vi "MagBoard_Processor.vi"() -> ()   [LabVIEW 2018]
uses:
  <vilib>/Math Plots/3D Math Plots/3D Surface/3D Surface XCtrl/3D Surface.xctl
  <vilib>/Math Plots/3D Math Plots/3D Surface/3D Surface Datatype/3D Surface Datatype.lvclass
  subVIs/calibration/FGVs/FGV States.ctl
  <vilib>/Utility/file.llb/Write Delimited Spreadsheet (DBL).vi
  <vilib>/Math Plots/3D Math Plots/3D Surface/3D Surface Datatype/Public/Plot Helper (Matrix).vi
panel:
  out "Node XYZ List":dbl[][](array[numeric])
  out "dT":u32=4294745741
  in  "Calibration File":string="6x0-5mm"
  in  "Save Data":bool=TRUE
  in  "Export File (CSV)":path=path "C:/Users/menprc/Documents/GitHub/MagLib/MagBoard_n64_UI/MagBoard_n64_UI_LabVIEW_Client/example_data/M064_008.csv"
  in  "dT":u32=10
  in  "Tare":bool
  out "Time":u32=4294745741
  in  "stop":bool
  in  "Data File":path=path "C:/Users/menprc/Documents/GitHub/MagLib/MagBoard_n64_UI/MagBoard_n64_UI_LabVIEW_Client/example_data/M064_008_up.dat"
  out "Instantaneous Data":refnum<class "3D Plot Datatype.lvclass">[](xcontrol)
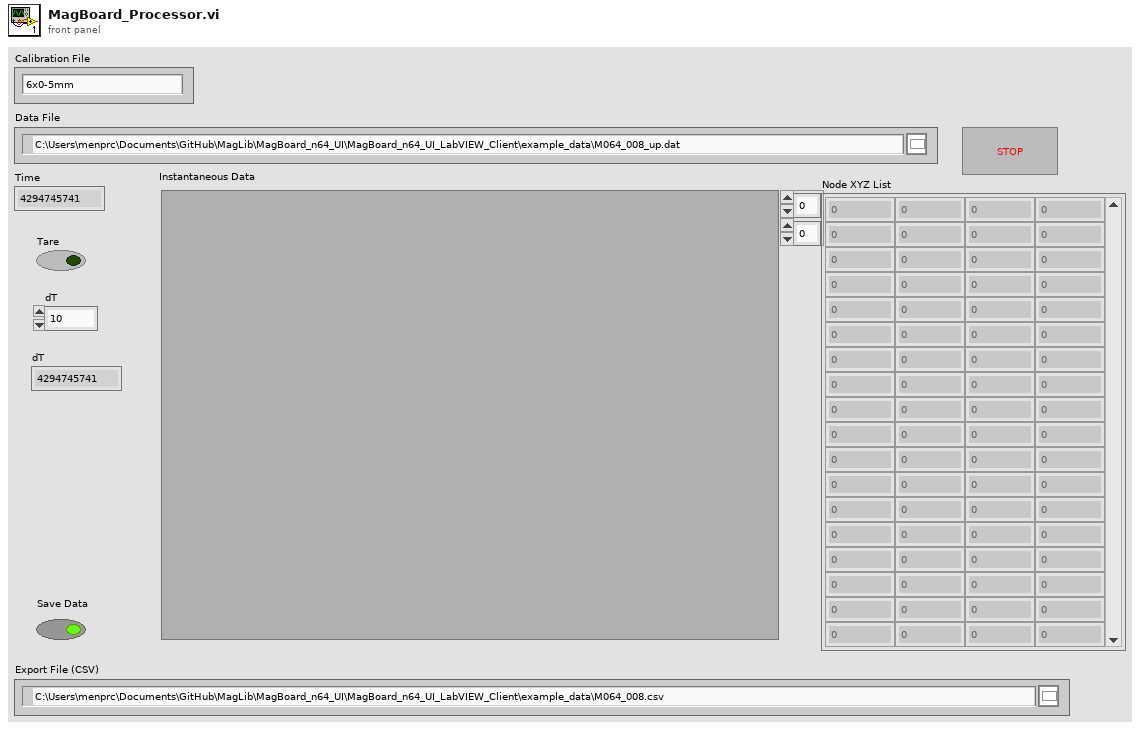
[diagram p1: front panel]
types:
  T1 = typedef "FGV States.ctl" = enum16{"Get", "Set", "Reset"}
  T2 = cluster{cluster{dbl[][], "Array":dbl[][]}, cluster{dbl[][], "Array":dbl[][]}, cluster{dbl[][], "Array":dbl[][]}, cluster{dbl[][], "Array":dbl[][]}}
  T3 = cluster{cluster{dbl[][], "Array":dbl[][]}, cluster{dbl[][], "Array":dbl[][]}, cluster{dbl[][], "Array":dbl[][]}, cluster{dbl[][], "Array":dbl[][]}}[]
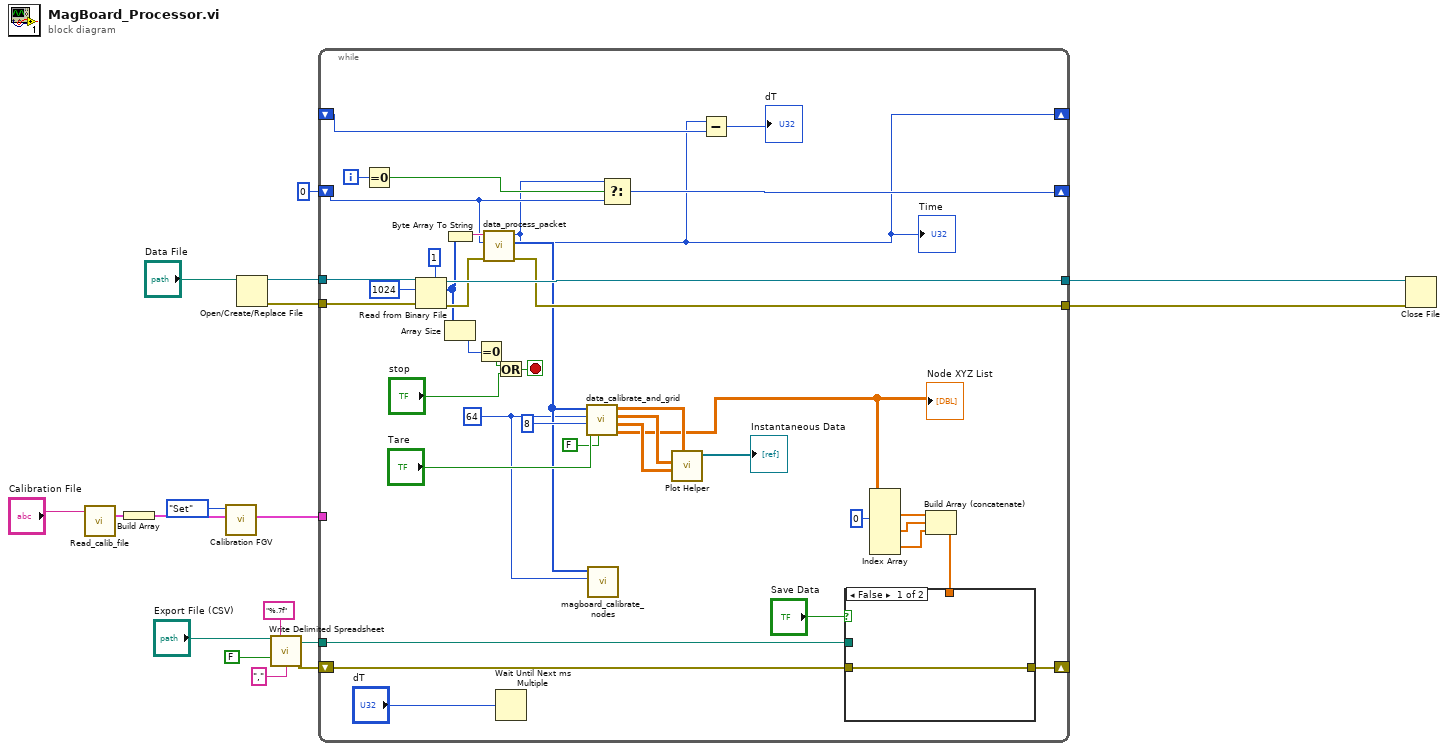
[diagram p0: block diagram]
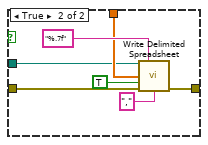
[diagram p2: hidden frame]
diagram:
  n1 = call "Read_calib_file.vi"("string"="Calibration File") -> ("output cluster"=w4:T2)  [unwired: 6 in, 4 out]
  n2 = Build Array(w4) -> (w3:T3)
  n3 = call "Calibration FGV.vi"("Calib in"=w3, "FGV States"=FGV_States."Set") -> ("Calib in 2"=w1:T3)  [unwired: 9 in]
  n4 = Open/Create/Replace File(file path (use dialog)="Data File") -> (refnum out=w16:refnum<file>, error out=w15:errorcluster)  [unwired: 5 in, 1 out]
  n5 = call-poly <vilib>:"Write Delimited Spreadsheet.vi"("file path (dialog if empty)"="Export File (CSV)", "format (%.3f)"="%.7f", "append to file? (new file:F)"=FALSE, "delimiter (\\t)"="," ("delimiter (\\t)")) -> ("new file path (Not A Path if cancelled)"=w8:path, "error out"=w6:errorcluster)  [unwired: 10 in]
  n6 = while {
    tunnel: w16 -> [w57]
    tunnel: w15 -> [w56]
    tunnel: [w54] -> w13
    tunnel: [w49] -> w14
    shift-right: [w48] -> _
    shift-left: u32 0 ("Time") -> [w46]
    tunnel: w8 -> [w32]
    shift-right: [w30] -> _
    shift-left: w6 -> [w31]
    tunnel: w1 -> [_]
    shift-right: [w19] -> _
    shift-left: _ -> [w20]
    i -> [w47]
    stop <- w25 stop-if-true
    w21 = 64 ("No. Nodes")
    n7 = Equal To 0?(x=w47) -> (x = 0?=w42:bool)
    n8 = Read from Binary File(5:u8 1 ("count (1)"), 8:w56, 10:1024 ("count (1)"), 11:w57) -> (0:w50:errorcluster, 2:w28:u8[], 3:w54:refnum<file>)  [unwired: 2 in, 1 out]
    n9 = Byte Array To String(unsigned byte array=w28) -> (string=w51:string)
    n10 = Array Size(array=w28) -> (size(s)=w27:i32)
    n11 = Equal To 0?(x=w27) -> (x = 0?=w26:bool)
    n12 = call "data_process_packet.vi"("error in (no error)"=w50, "No. Sensors"=w46, "Binary Input Data"=w51) -> ("error out"=w49:errorcluster, "Raw Sensors (Flattened)"=w22:i16[], "Time"=w19:u32)  [unwired: 4 in, 2 out]
    "Time" <- w19
    n13 = Or(x=w26, y="stop") -> (x .or. y?=w25:bool)
    n14 = Wait Until Next ms Multiple(millisecond multiple="dT") -> ()  [unwired: 1 out]
    n15 = call "data_calibrate_and_grid.vi"("Reset"=FALSE, "Tare"="Tare", "Row Length"=8, "No. Nodes"=w21, "Sensor Readings (PACKET)"=w22) -> ("Node XYZ List"=w23:dbl[][], "Y (GRID)"=w40:dbl[][], "X (GRID)"=w41:dbl[][], "Z (GRID)"=w43:dbl[][])  [unwired: 2 in, 1 out]
    "Node XYZ List" <- w23
    n16 = call "magboard_calibrate_nodes.vi"("No. Nodes"=w21, "Sensor Readings (PACKET)"=w22) -> ()  [unwired: 9 in, 1 out]
    n17 = Select(t=w19, s=w42, f=w46) -> (s? t:f=w48:u32)
    n18 = call-poly <vilib>:"Plot Helper.vi"("z matrix"=w43, "y matrix"=w40, "x matrix"=w41) -> ("3D Plot lvclass Array out"=→"Instantaneous Data":refnum<class "3D Plot Datatype.lvclass">[])  [unwired: 3 in, 5 out]
    n19 = Subtract(x=w19, y=w20) -> (x-y=→"dT":u32)
    n20 = Index Array(array=w23, index (col) #1=0 ("disabled index (col)")) -> (element #1=w36:dbl[], element #2=w35:dbl[], element #3=w34:dbl[])  [unwired: 5 in]
    n21 = Build Array (concatenate)(w36, w35, w34) -> (w33:dbl[])
    n22 = case shown="False" "Save Data" {
      tunnel: w33 -> [_ w62]
      tunnel: w32 -> [_ w61]
      tunnel: w31 -> [w58 w60]
      tunnel: [w58 w59] -> w30
      frame False {
      }
      frame True {
        n23 = call-poly <vilib>:"Write Delimited Spreadsheet.vi"("file path (dialog if empty)"=w61, "format (%.3f)"="%.7f", "1D data"=w62, "append to file? (new file:F)"=TRUE, "error in (no error)"=w60, "delimiter (\\t)"="," ("delimiter (\\t)")) -> ("error out"=w59:errorcluster)  [unwired: 8 in, 1 out]
      }
    }
  }
  n24 = Close File(refnum=w13, error in=w14) -> ()  [unwired: 2 out]
